vi "XLP80_Action_EnableCVMTestmode_A.vi"(7 "but_Enable reading cell voltage":bool caption="Enable reading cell voltage", 8 "err in":errorcluster) -> (0 "err out":errorcluster)   [LabVIEW 2021]
uses:
  XLP80_FGlob/1886_FGlob_TDefs_Enum_FGlobItems.ctl
  XLP80_FGlob/1886_FGlob_TDefEnumCANWriteItems.ctl
  XLP80_Globals/XLP80_Globals_Referenzen.vi
  XLP80_Globals/XLP80_CAN_Globals.vi
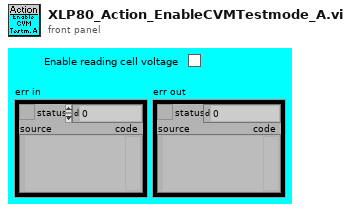
[diagram p1: front panel]
types:
  T1 = typedef "1886_FGlob_TDefs_Enum_FGlobItems.ctl" = enum16{"Put one", "Put all", "Recall one", "Recall all"}
  T2 = typedef "1886_FGlob_TDefEnumCANWriteItems.ctl" = enum16{"LV_Testmode_Select", "LV_A_71_Current_Out_Set", "LV_A_71_Voltage_In_Set", "LV_A_71_Voltage_Out_Set", "LV_H_51_STK_CellVoltages_Enable", "S80_BP_s_Taster_Start_Status"}
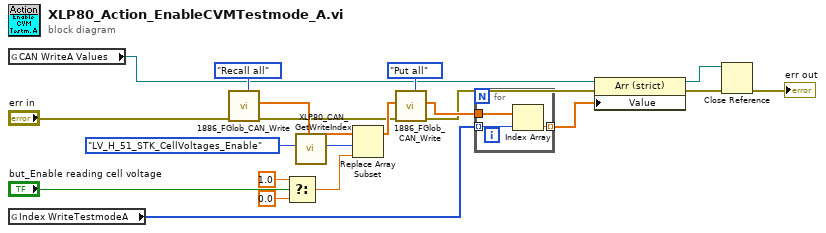
[diagram p0: block diagram]
diagram:
  n1 = global read "XLP80_Globals_Referenzen.vi" "CAN WriteA Values"() -> (w6:refnum<vi>)
  n2 = global read "XLP80_CAN_Globals.vi" "Index WriteTestmodeA"() -> (w19:i32[])
  n3 = call "1886_FGlob_CAN_Write.vi"("Function (Recall One)"=1886_FGlob_TDefs_Enum_FGlobItems."Recall all", "err in"="err in") -> ("err out"=w12:errorcluster, "AO Values OUT"=w14:dbl[])  [unwired: 7 in, 1 out]
  n4 = Select(t=1.0 ("new element/subarray"), s="but_Enable reading cell voltage", f=0.0 ("new element/subarray")) -> (s? t:f=w1:dbl)
  n5 = call "XLP80_CAN_GetWriteIndex.vi"("CAN Write Items"=1886_FGlob_TDefEnumCANWriteItems."LV_H_51_STK_CellVoltages_Enable" ("CAN Write Items Testmode_A")) -> ("Index"=w17:i32)  [unwired: 10 in]
  n6 = Replace Array Subset(array=w14, new element=w1, index=w17) -> (w13:dbl[])
  n7 = call "1886_FGlob_CAN_Write.vi"("Function (Recall One)"=1886_FGlob_TDefs_Enum_FGlobItems."Put all", "err in"=w12, "AO Values IN"=w13) -> ("err out"=w9:errorcluster, "AO Values OUT"=w11:dbl[])  [unwired: 6 in, 1 out]
  n8 = for {
    tunnel: w19 -> [w22] mode=indexing
    tunnel: w11 -> [w23]
    tunnel: [w21] -> w10 mode=indexing
    n9 = Index Array(array=w23, index=w22) -> (element=w21:dbl)
  }
  n10 = property class="Arr (strict)"(reference=w6, error in=w9, "Value"=w10) -> (reference out=w7:refnum<vi>, error out=w8:errorcluster)
  n11 = Close Reference(reference=w7, error in (no error)=w8) -> (error out=→"err out":errorcluster)
